vi "EXPORT LISTBOX TO CLIPBOARD.vi"(11 "LISTBOX REFERENCE IN":refnum<vi>) -> ()   [LabVIEW 2019]
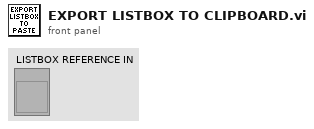
[diagram p1: front panel]
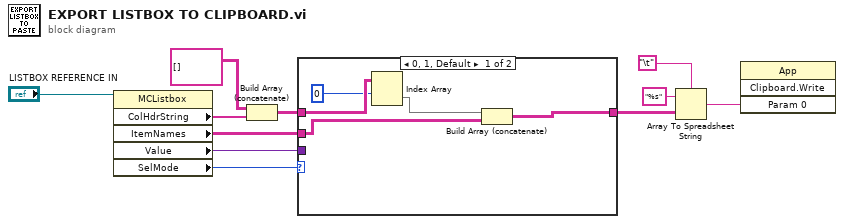
[diagram p0: block diagram]
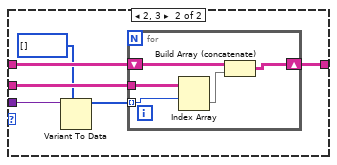
[diagram p2: hidden frame]
diagram:
  n1 = property class="MCListbox"(reference="LISTBOX REFERENCE IN") -> ("ColHdrString"=w7:string[], "ItemNames"=w10:string[][], "Value"=w9:variant, "SelMode"=w2:i32)  [unwired: 1 in, 2 out]
  n2 = Build Array (concatenate)(string[][] [], w7) -> (w6:string[][])
  n3 = case shown="0, 1, Default" w2 {
    tunnel: w10 -> [w15 w22]
    tunnel: w9 -> [_ w19]
    tunnel: w6 -> [w14 w21]
    tunnel: [w16 w20] -> w5
    frame 0, 1, Default {
      n4 = Index Array(array=w14, index (row)=0 ("Search Database Results")) -> (element=w12:string[])  [unwired: 1 in]
      n5 = Build Array (concatenate)(w12, w15) -> (w16:string[][])
    }
    frame 2, 3 {
      n6 = Variant To Data(type=i32[] [] ("User's Checked Out Items"), Variant=w19) -> (data=w17:i32[])  [unwired: 1 in, 1 out]
      n7 = for {
        tunnel: w17 -> [w25] mode=indexing
        shift-right: [w23] -> w20
        shift-left: w21 -> [w27]
        tunnel: w22 -> [w26]
        n8 = Index Array(array=w26, index (row)=w25) -> (element=w24:string[])  [unwired: 1 in]
        n9 = Build Array (concatenate)(w27, w24) -> (w23:string[][])
      }
    }
  }
  n10 = Array To Spreadsheet String(delimiter (Tab)="\t", array=w5, 3:"%s" ("format string")) -> (spreadsheet string=w4:string)
  n11 = invoke class="App" method="Clipboard.Write"("Param 0"=w4) -> ()  [unwired: 3 in, 4 out]
